vi "Match.vi"(10 "log record":T1 {"timestamp" format="%<%x %.3X>T"}, 11 "combination filter":refnum<class "Combination.lvclass">) -> (2 "matches?":bool[](array[boolean]), 3 "dup combination filter":refnum<class "Combination.lvclass">)   [LabVIEW 2018, in "GLog.lvlib" / "Combination.lvclass"]
uses:
  Combination.lvclass
  Log Record.ctl
  logger_class/Internal Log Levels.ctl
  Combination.lvclass/Combination.ctl
  extension/filter_interface/Filter.lvclass
  GLog.lvlib
panel:
  # "Connector Pane"
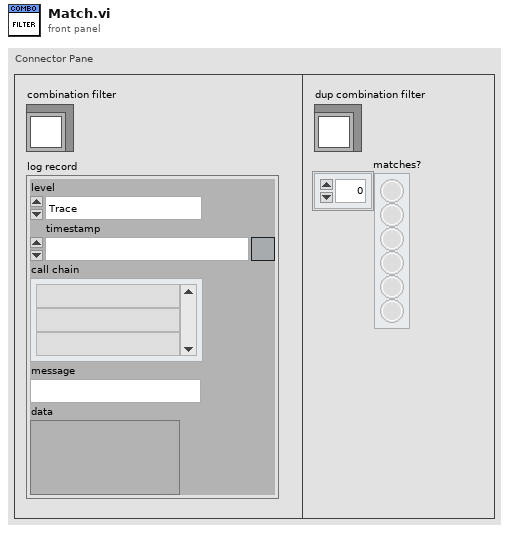
[diagram p1: front panel]
types:
  T1 = typedef "GLog.lvlib/Log Record.ctl" = cluster{"level":T2, "timestamp":timestamp, "call chain":string[], "message":string, "data":variant}
  T2 = typedef "GLog.lvlib/Internal Log Levels.ctl" = enum16{"Trace", "Debug", "Info", "Warning", "Error", "Critical", "Internal"}
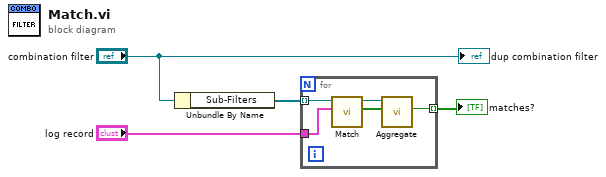
[diagram p0: block diagram]
diagram:
  n1 = Unbundle By Name("combination filter") -> ("Sub-Filters"=w4:refnum<class "Filter.lvclass">[])
  n2 = for {
    tunnel: w4 -> [w9] mode=indexing
    tunnel: "log record" -> [w8]
    tunnel: [w6] -> w1 mode=indexing
    n3 = call-dynamic "Match.vi"("log record"=w8, "filter in"=w9) -> ("matches"=w7:bool[], "filter out"=w5:refnum<class "Filter.lvclass">)  [unwired: 8 in]
    n4 = call "Aggregate.vi"("matches"=w7, "filter"=w5) -> ("match?"=w6:bool)  [unwired: 8 in, 1 out]
  }
  "matches?" <- w1
  "dup combination filter" <- "combination filter"
